vi "GetColorScaleReference.vi"(8 "error in":errorcluster, 11 "ColorScale in":refnum<class "ColorScale.lvclass">) -> (0 "error out":errorcluster, 1 "color scale reference":refnum<vi>, 3 "ColorScale out":refnum<class "ColorScale.lvclass">)   [LabVIEW 2014, in "ColorScale.lvclass"]
uses:
  ColorScale.lvclass
  Generic/Generic.lvclass
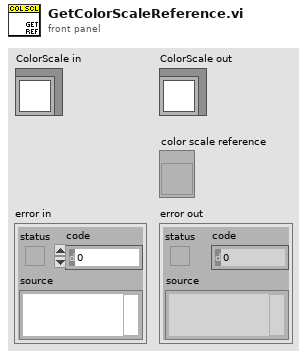
[diagram p1: front panel]
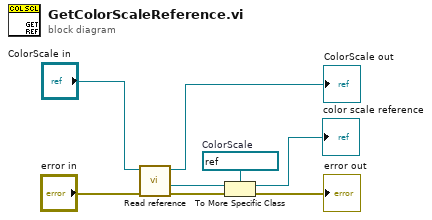
[diagram p0: block diagram]
diagram:
  w5 = refnum<vi> refnum  # ColorScale
  n1 = call "Read reference.vi"("error in"="error in", "GObject in"="ColorScale in") -> ("error out"=w6:errorcluster, "reference"=w7:refnum<vi>, "GObject out"=→"ColorScale out":refnum<class "ColorScale.lvclass">)  [unwired: 5 in]
  n2 = To More Specific Class(target class=w5, reference=w7, error in=w6) -> (specific class reference=→"color scale reference":refnum<vi>, error out=→"error out":errorcluster)
